vi "Write MFC.vi"(8 "error in (no error)":errorcluster, 11 "MFC in":refnum<class "MFC.lvclass">) -> (0 "error out":errorcluster, 3 "MFC out":refnum<class "MFC.lvclass">)   [LabVIEW 2013, in "MFC.LVLIB" / "MFC.lvclass"]
uses:
  MFC.lvclass
  <vilib>/Instr/_visa.llb/VISA Flush IO Buffer Mask.ctl
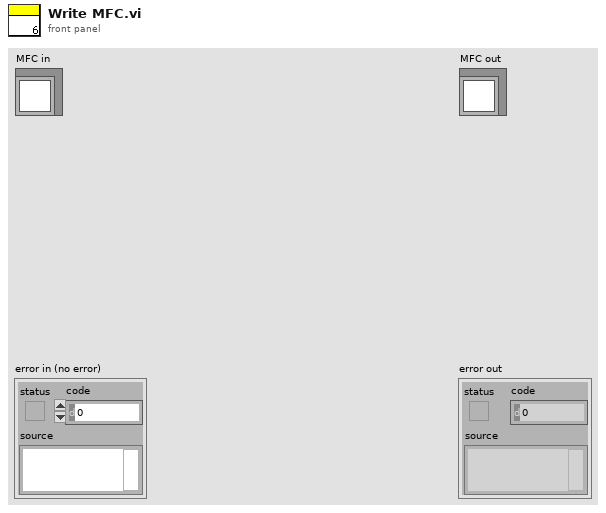
[diagram p1: front panel]
types:
  T1 = typedef "VISA Flush IO Buffer Mask.ctl" = u16
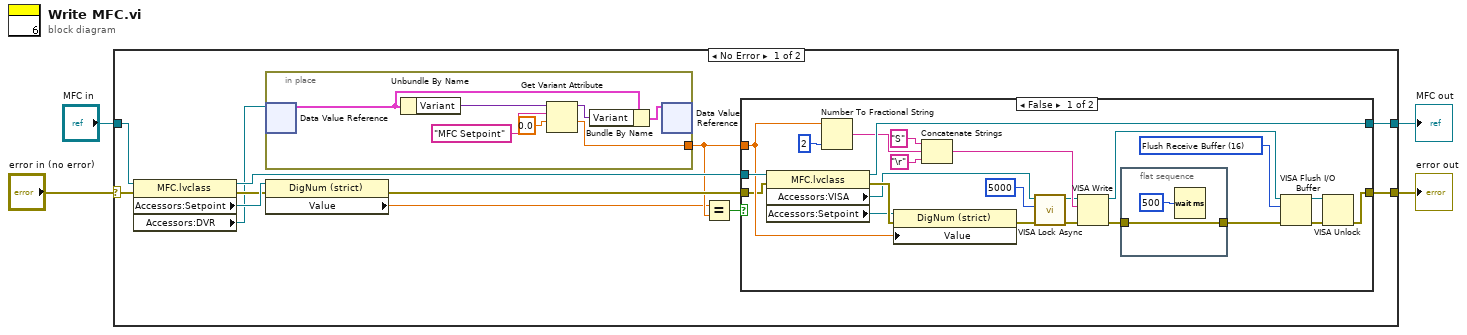
[diagram p0: block diagram]
diagram:
  n1 = case shown="No Error" "error in (no error)" {
    selector: "error in (no error)" -> [w15 w52]
    tunnel: [w5 w52] -> w1
    tunnel: [w6 w51] -> w2
    tunnel: "MFC in" -> [w16 w51]
    frame No Error {
      n2 = property class="MFC.lvclass"(reference=w16, error in=w15) -> (reference out=w14:refnum<class "MFC.lvclass">, error out=w12:errorcluster, "Accessors:Setpoint"=w13:refnum<vi>, "Accessors:DVR"=w7:refnum<data-value>)
      n3 = in-place {
        in-place-border: [w44] -> w9
        n4 = in-place-dvr #1(w7) -> (w47:cluster{"Array":string[], "Variant":variant})  [unwired: 1 out]
        n5 = Unbundle By Name(w47) -> ("Variant"=w49:variant)
        n6 = Get Variant Attribute(Variant=w49, name="MFC Setpoint", default value (empty Variant)=0.0) -> (duplicate Variant=w48:variant, value=w44:dbl)  [unwired: 1 in, 2 out]
        n7 = Bundle By Name(cluster=w47, "Variant"=w48) -> (w50:cluster{"Array":string[], "Variant":variant})
        n8 = in-place-dvr #1(w50) -> ()  [unwired: 2 out]
      }
      n9 = property class="DigNum (strict)"(reference=w13, error in=w12) -> (error out=w11:errorcluster, "Value"=w8:dbl)  [unwired: 1 out]
      n10 = Equal?(x=w8, y=w9) -> (x = y?=w10:bool)
      n11 = case shown="False" w10 {
        tunnel: w14 -> [w39 w43]
        tunnel: [w17 w42] -> w5
        tunnel: [w38 w43] -> w6
        tunnel: w9 -> [w27 _]
        tunnel: w11 -> [w26 w42]
        frame False {
          w29 = T1 16 items=["Flush Receive Buffer"=16, "Write Transmit Buffer to Device"=32, "Flush Receive Buffer (No I/O)"=64, "Flush Transmit Buffer"=128] ("Mask")
          n12 = property class="MFC.lvclass"(reference=w39, error in=w26) -> (reference out=w38:refnum<class "MFC.lvclass">, error out=w28:errorcluster, "Accessors:VISA"=w22:refnum<visa-resource-name>, "Accessors:Setpoint"=w25:refnum<vi>)
          n13 = Number To Fractional String(number=w27, precision (6)=i16 2) -> (F-format string=w35:string)  [unwired: 2 in]
          n14 = property class="DigNum (strict)"(reference=w25, error in=w28, "Value"=w27) -> (error out=w24:errorcluster)  [unwired: 1 out]
          n15 = Concatenate Strings("S" ("string"), w35, "\r") -> (w32:string)
          n16 = call <vilib>:"VISA Lock Async.vi"("error in (no error)"=w24, "timeout (0)"=u32 5000, "VISA resource name"=w22) -> ("error out"=w23:errorcluster, "VISA resource name out"=w21:refnum<visa-resource-name>)  [unwired: 6 in, 1 out]
          n17 = VISA Write(VISA resource name=w21, write buffer=w32, error in (no error)=w23) -> (VISA resource name out=w30:refnum<visa-resource-name>, error out=w37:errorcluster)  [unwired: 1 out]
          n18 = flat-sequence {
            tunnel: [w40] -> w31
            tunnel: w37 -> [w40]
            frame #0 {
              n19 = Wait (ms)(milliseconds to wait=u32 500) -> ()  [unwired: 1 out]
            }
          }
          n20 = VISA Flush I/O Buffer(VISA resource name=w30, mask (16)=w29, error in (no error)=w31) -> (VISA resource name out=w19:refnum<visa-resource-name>, error out=w18:errorcluster)
          n21 = VISA Unlock(8:w18, 11:w19) -> (0:w17:errorcluster)  [unwired: 1 out]
        }
        frame True {
        }
      }
    }
    frame Error {
    }
  }
  "error out" <- w1
  "MFC out" <- w2
